vi "QD_Store_100.vi"(0 "Generated_Data_In":T1, 1 "Max_Queue_Size_In":i32=-1, 2 "Queue_Name_In":string, 5 "Time_Out_In_ms (-1)":i32=-1, 11 "Error_In":errorcluster, 13 "Queue_Operation":T2=enum."Flush") -> (4 "Generated_Data_Out":T1, 6 "Total_Data":T1[](array[typedef]), 15 "Error_Out":errorcluster)   [LabVIEW 2023]
doc: "Used to transfer data from one vi to another using queue."
uses:
  Controls/Queue_Operation_Select.ctl
  Controls/Generated_data.ctl
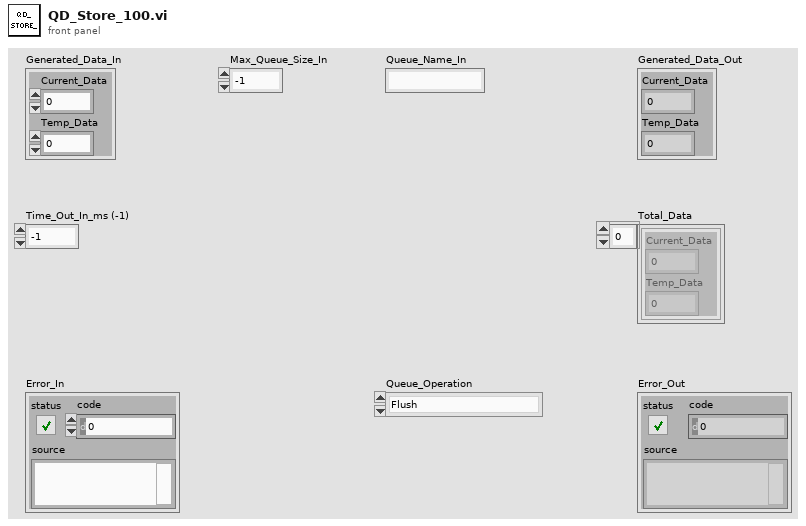
[diagram p1: front panel]
types:
  T1 = typedef "Generated_data.ctl" = cluster{"Current_Data":dbl, "Temp_Data":dbl}
  T2 = typedef "Queue_Operation_Select.ctl" = enum16{"Obtain_Queue", "Enqueue", "Enqueue_N", "Lossy_Enqueue", "Preview", "Queue_Status", "Release_Queue", "Dequeue", "Flush"}
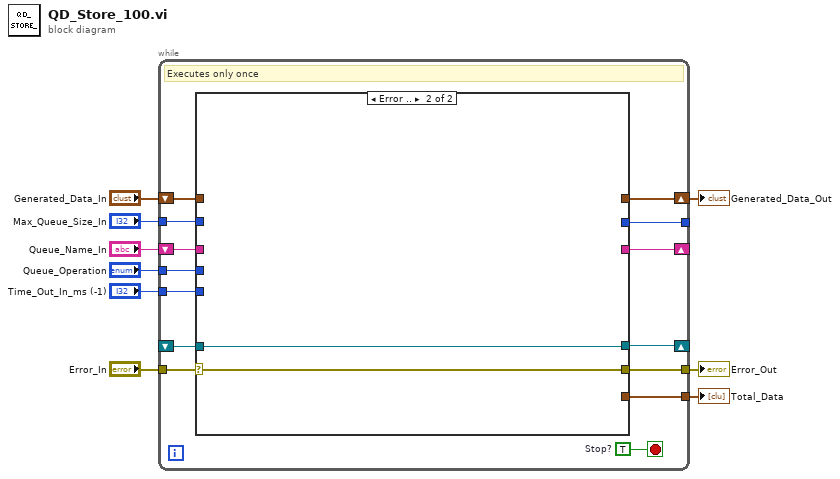
[diagram p0: block diagram]
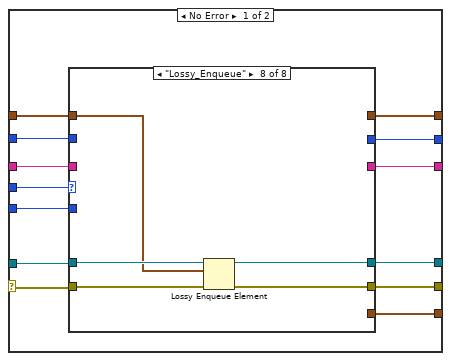
[diagram p2: hidden frame]
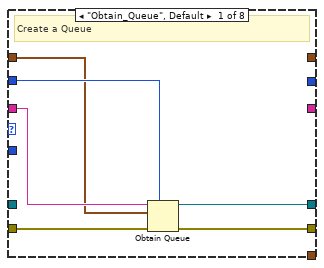
[diagram p3: hidden frame]
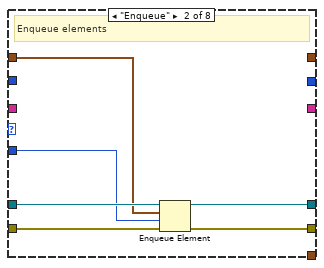
[diagram p4: hidden frame]
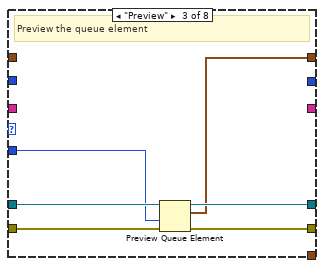
[diagram p5: hidden frame]
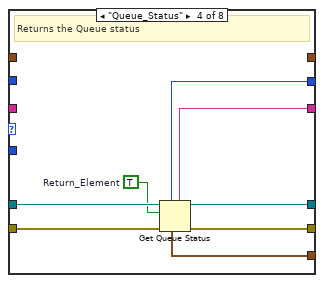
[diagram p6: hidden frame]
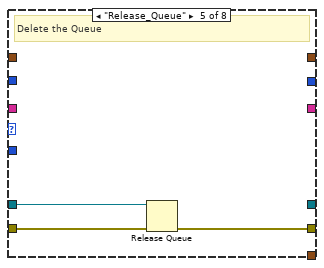
[diagram p7: hidden frame]
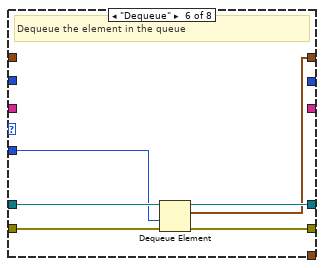
[diagram p8: hidden frame]
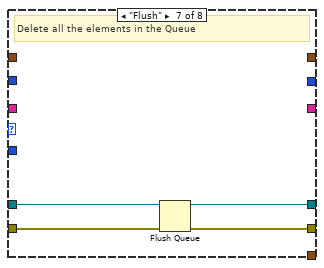
[diagram p9: hidden frame]
diagram:
  n1 = while {
    tunnel: "Max_Queue_Size_In" -> [w23]
    tunnel: "Time_Out_In_ms (-1)" -> [w20]
    tunnel: [w18] -> _
    tunnel: "Queue_Operation" -> [w15]
    tunnel: [w13] -> w2
    shift-right: [w19] -> w1
    shift-left: "Generated_Data_In" -> [w21]
    shift-right: [w17] -> _
    shift-left: "Queue_Name_In" -> [w14]
    shift-right: [w16] -> _
    shift-left: _ -> [w11]
    tunnel: "Error_In" -> [w12]
    tunnel: [w22] -> w8
    stop <- w10 stop-if-true
    w10 = TRUE  # Stop?
    # "Executes only once"
    n2 = case shown="Error .." w12 {
      selector: w12 -> [w25 w82]
      tunnel: w15 -> [w26 _]
      tunnel: w14 -> [w27 _]
      tunnel: w23 -> [w36 _]
      tunnel: [w35 w81] -> w16
      tunnel: [w34 w82] -> w22
      tunnel: w21 -> [w28 _]
      tunnel: w20 -> [w33 _]
      tunnel: [w32 _] -> w19
      tunnel: [w31 _] -> w18
      tunnel: [w30 _] -> w17
      tunnel: [w29 _] -> w13
      tunnel: w11 -> [w24 w81]
      frame No Error {
        n3 = case shown="\"Lossy_Enqueue\"" w26 {
          tunnel: w25 -> [w42 w48 w53 w61 w64 w70 w74 w79]
          tunnel: w27 -> [w40 _ _ _ _ _ _ _]
          tunnel: w36 -> [w39 _ _ _ _ _ _ _]
          tunnel: [w37 w44 w52 w60 _ w69 w73 w78] -> w35
          tunnel: [w41 w47 w51 w59 w63 w67 w72 w77] -> w34
          tunnel: w24 -> [_ w46 w54 w62 w65 w71 w75 w80]
          tunnel: w28 -> [w38 w45 _ _ _ _ _ w76]
          tunnel: w33 -> [_ w43 w50 _ _ w66 _ _]
          tunnel: [_ _ w49 _ _ w68 _ _] -> w32
          tunnel: [_ _ _ w58 _ _ _ _] -> w31
          tunnel: [_ _ _ w57 _ _ _ _] -> w30
          tunnel: [_ _ _ w56 _ _ _ _] -> w29
          frame "Obtain_Queue", Default {
            # "Create a Queue"
            n4 = Obtain Queue(max queue size (-1, unlimited)=w39, name (unnamed)=w40, element data type=w38, error in (no error)=w42) -> (queue out=w37:refnum<queue>, error out=w41:errorcluster)  [unwired: 1 in, 1 out]
          }
          frame "Enqueue" {
            # "Enqueue elements"
            n5 = Enqueue Element(queue=w46, element=w45, timeout in ms (-1)=w43, error in (no error)=w48) -> (queue out=w44:refnum<queue>, error out=w47:errorcluster)  [unwired: 1 out]
          }
          frame "Preview" {
            # "Preview the queue element"
            n6 = Preview Queue Element(queue=w54, timeout in ms (-1)=w50, error in (no error)=w53) -> (queue out=w52:refnum<queue>, element=w49:T1, error out=w51:errorcluster)  [unwired: 1 out]
          }
          frame "Queue_Status" {
            w55 = TRUE  # Return_Element
            # "Returns the Queue status"
            n7 = Get Queue Status(queue=w62, return elements? (F)=w55, error in (no error)=w61) -> (queue out=w60:refnum<queue>, queue name=w57:string, max queue size=w58:i32, error out=w59:errorcluster, elements=w56:T1[])  [unwired: 3 out]
          }
          frame "Release_Queue" {
            # "Delete the Queue"
            n8 = Release Queue(queue=w65, error in (no error)=w64) -> (error out=w63:errorcluster)  [unwired: 1 in, 2 out]
          }
          frame "Dequeue" {
            # "Dequeue the element in the queue"
            n9 = Dequeue Element(queue=w71, timeout in ms (-1)=w66, error in (no error)=w70) -> (queue out=w69:refnum<queue>, element=w68:T1, error out=w67:errorcluster)  [unwired: 1 out]
          }
          frame "Flush" {
            # "Delete all the elements in the Queue"
            n10 = Flush Queue(queue=w75, error in (no error)=w74) -> (queue out=w73:refnum<queue>, error out=w72:errorcluster)  [unwired: 1 out]
          }
          frame "Lossy_Enqueue" {
            n11 = Lossy Enqueue Element(queue=w80, element=w76, error in (no error)=w79) -> (queue out=w78:refnum<queue>, error out=w77:errorcluster)  [unwired: 2 out]
          }
        }
      }
      frame Error {
      }
    }
  }
  "Error_Out" <- w8
  "Total_Data" <- w2
  "Generated_Data_Out" <- w1
